vi "calibrationElectrometer_monitorCommand_StopScan.vi"(8 "error in (no error)":errorcluster, 11 "command_StopScan_Ctl":T1) -> (0 "error out":errorcluster, 2 "function return":i32, 3 "command_StopScan_Ctl out":T1)   [LabVIEW 2016, in "SALLV_calibrationElectrometer.lvlib"]
doc: "int calibrationElectrometer_shm_monitorCommand_StopScanLV(calibrationElectrometer_command_StopScanLV *command_StopScan_Ctl );"
uses:
  SALLV_calibrationElectrometer.lvlib
  DataTypes/command_StopScan.ctl
  SALLV_calibrationElectrometer.so
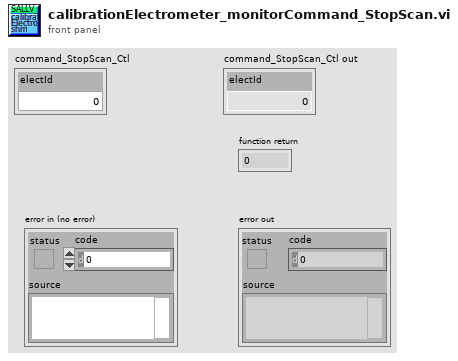
[diagram p1: front panel]
types:
  T1 = typedef "SALLV_calibrationElectrometer.lvlib/command_StopScan.ctl" = cluster{"electId":i16}
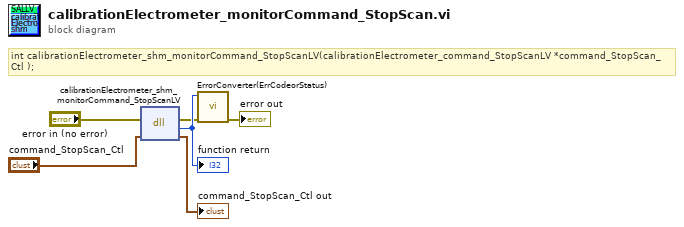
[diagram p0: block diagram]
diagram:
  # "int calibrationElectrometer_shm_monitorCommand_StopScanLV(calibrationElectrometer_command_StopScanLV *command_StopScan_Ctl );"
  n1 = dll-call lib="home/saluser/Desktop/SAL_Electrometer/SALLV_calibrationElectrometer.*" fn="calibrationElectrometer_shm_monitorCommand_StopScanLV"(error in="error in (no error)", "command_StopScan_Ctl"="command_StopScan_Ctl") -> (error out=w2:errorcluster, w6:i32, "command_StopScan_Ctl"=→"command_StopScan_Ctl out":T1)  [unwired: 2 in, 1 out]
  "function return" <- w6
  n2 = call "ErrorConverter(ErrCodeorStatus).vi"("error in (no error)"=w2, "error code"=w6) -> ("error out"=→"error out":errorcluster)  [unwired: 9 in]
